vi "GUI_Bella_EnergyChart.vi"() -> ()   [LabVIEW 2013]
uses:
  Shared/GUI_Template/GUI_master/tcp_new_data_event.ctl
  Shared/GUI_Template/GUI_master/tcp new data cluster.ctl
panel:
  out "Numeric 2":dbl format="%#_4g"
  out "Numeric":dbl format="%#_4g"
  out "Numeric 4":dbl format="%#_4g"
  out "Numeric 3":dbl format="%#_4g"
  out "Numeric 7":dbl format="%#_4g"
  out "Numeric 9":dbl format="%#_4g"
  out "Numeric 5":dbl format="%#_4g"
  out "Numeric 6":dbl format="%#_4g"
  out "Numeric 8":dbl format="%#_4g"
  out "Numeric 10":dbl format="%#_4g"
  out "Numeric 11":dbl format="%#_4g"
  out "Numeric 12":dbl format="%#_4g"
  out "Numeric 13":dbl format="%#_4g"
  out "Numeric 14":dbl format="%#_4g"
  in  "stop":bool
  in  "RawField::1":dbl=0.001 caption="Raw Field" min=0.0 max=0.0 format="%_4f"
  in  "field::1":dbl=0.001 caption="Field" min=0.0 max=0.0 format="%_4p"
  in  "GUIdevice 1":string="BELLA_HallProbe"
  out "tcp data event":T1
  out "error IO 2":errorcluster
  # "Energy Chart"
  # "cam1"
  # "cam2"
  # "High Energy screen"
  # "[MeV/c]"
  # "Mid Energy screen"
  # "cam3"
  # "cam4"
  # "cam5"
  # "[MeV/c]"
  # "cam6"
  # "cam7"
  # "cam8"
  # "cam9"
  # "cam10"
  # "cam11"
  # "cam12"
  # "[MeV/c]"
  # "Low Energy screen, cam6 - 12"
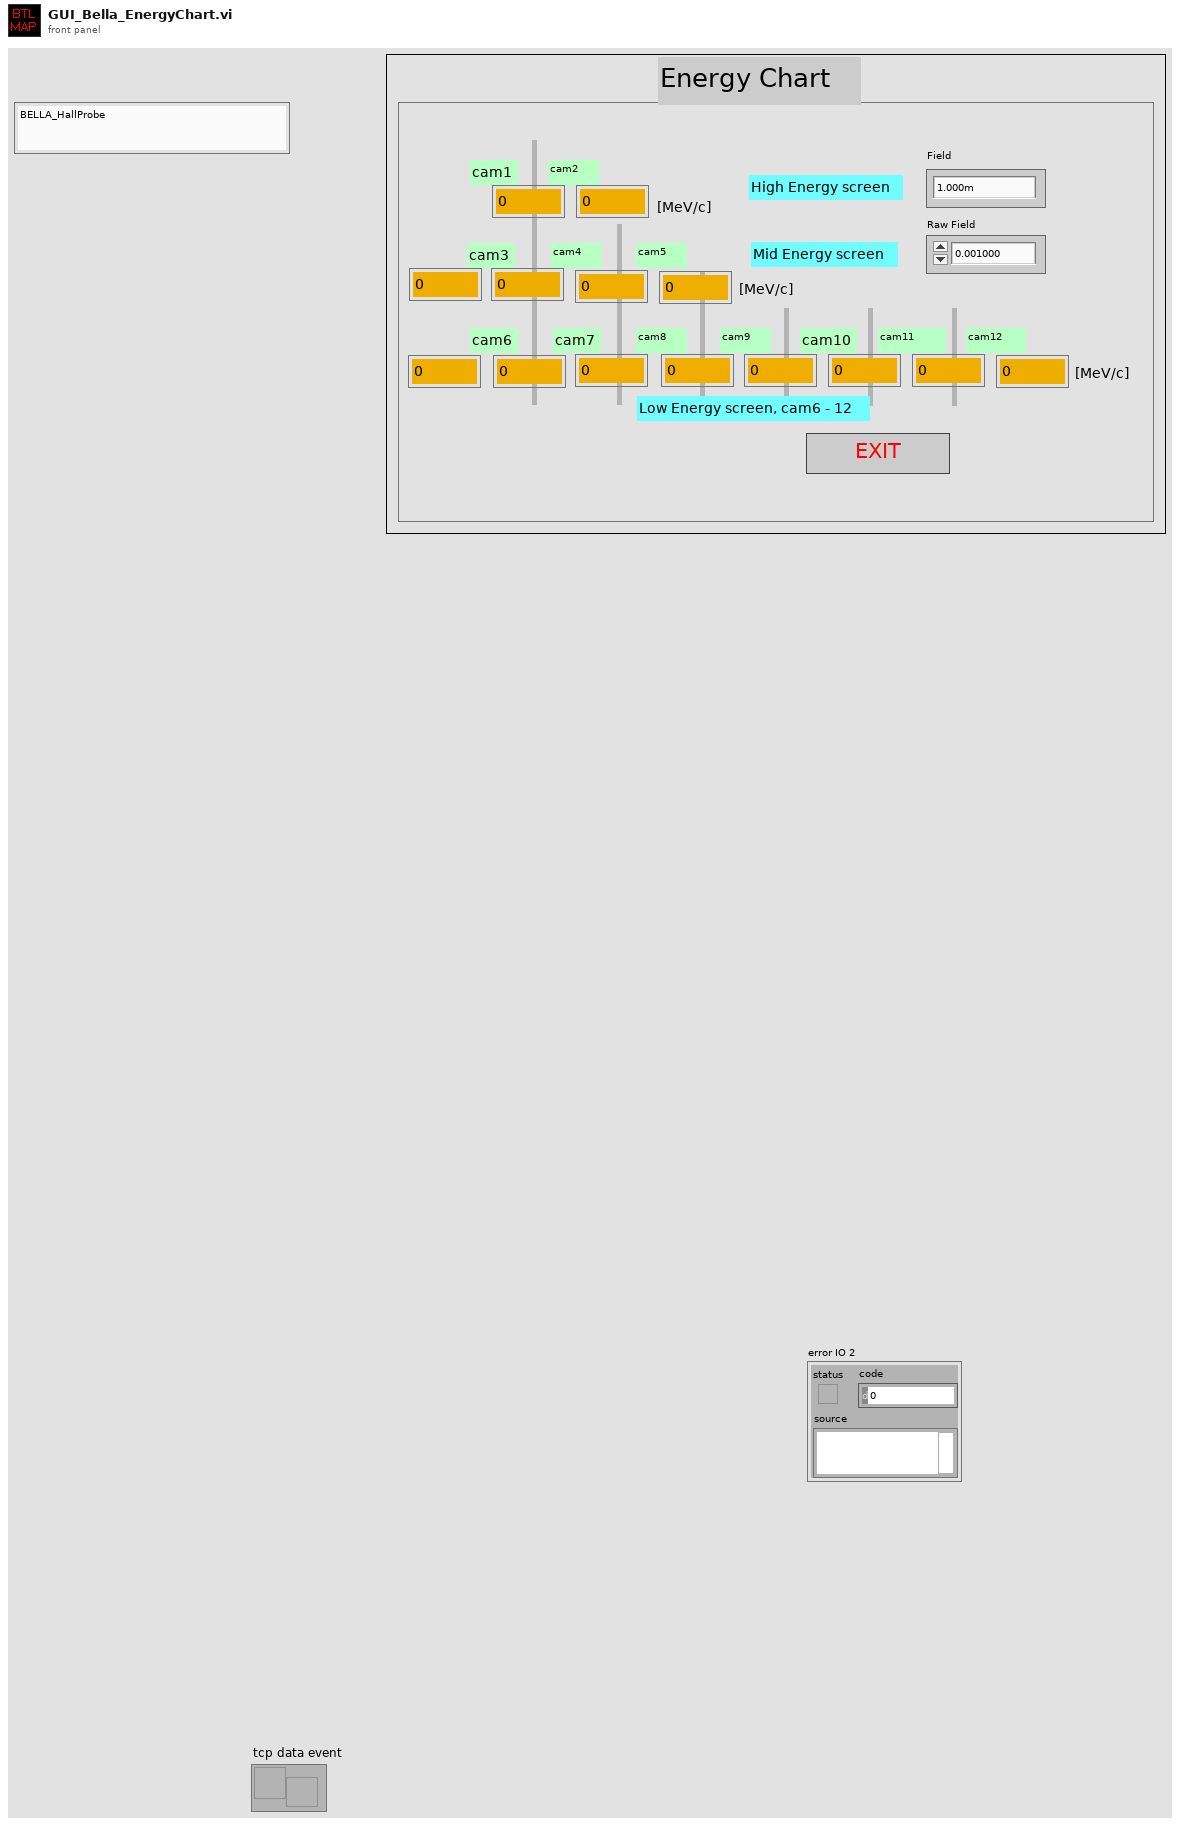
[diagram p1: front panel]
types:
  T1 = typedef "tcp_new_data_event.ctl" = refnum<user-event>
  T2 = typedef "tcp new data cluster.ctl" = cluster{"EventEnum":enum16{"new data", "connection status update"}, "Device name":string}
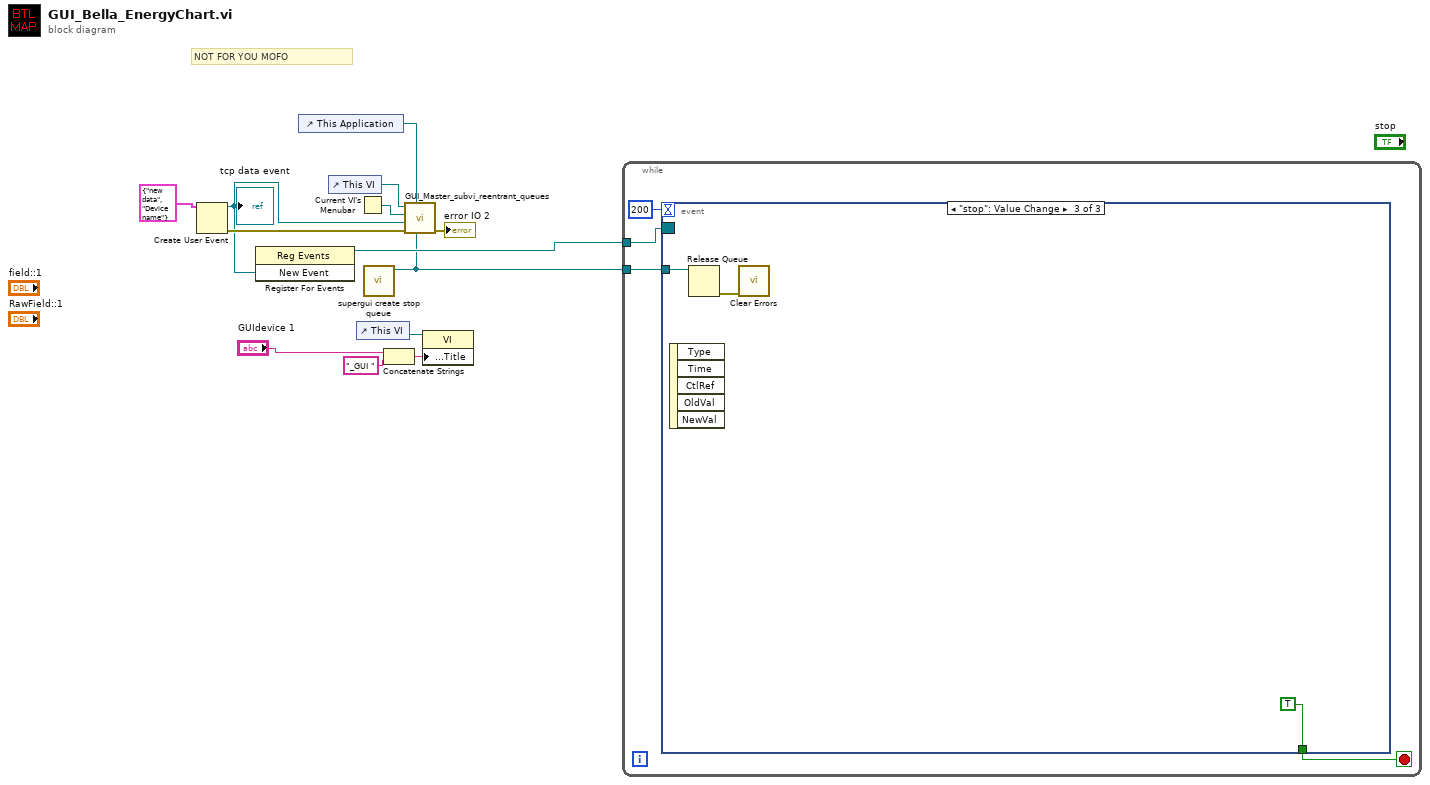
[diagram p0: block diagram]
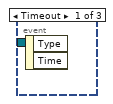
[diagram p2: hidden frame]
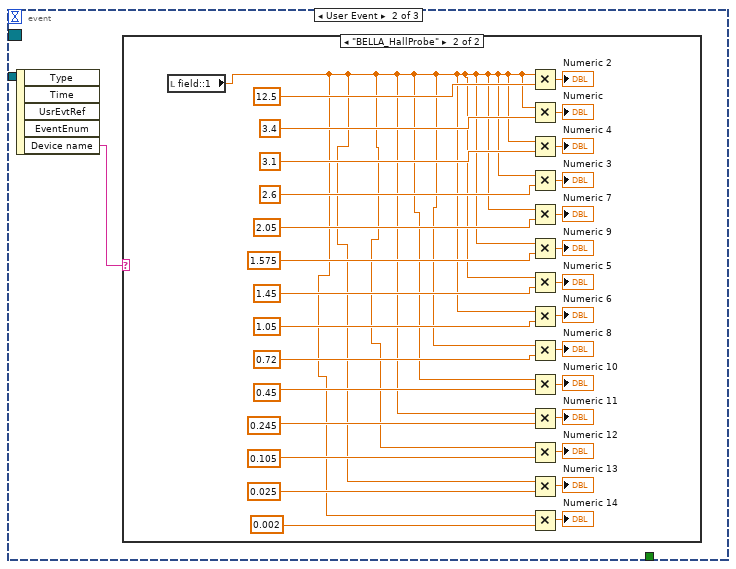
[diagram p3: hidden frame]
diagram:
  # "NOT FOR YOU MOFO"
  n1 = Create User Event(user event datatype=T2 {"EventEnum"=enum."new data", "Device name"="Device name"} ("New Event")) -> (user event=w8:refnum<user-event>, error out=w9:errorcluster)  [unwired: 1 in]
  "tcp data event" <- w8
  n2 = register-events(w8) -> (reference out=w6:refnum<event-registration>)  [unwired: 2 in, 1 out]
  n3 = control-ref of="This Application"() -> (w7:refnum<vi>)
  n4 = control-ref of="This VI"() -> (w12:refnum<vi>)
  n5 = control-ref of="This VI"() -> (w4:refnum<vi>)
  n6 = Current VI's Menubar() -> (w11:refnum<k9>)
  n7 = call "supergui create stop queue.vi"() -> ("STOP Queue out"=w5:refnum<queue>)  [unwired: 11 in]
  n8 = Concatenate Strings("GUIdevice 1", "_GUI ") -> (w3:string)
  n9 = call "GUI_Master_subvi_reentrant_queues.vi"("STOP Queue in"=w5, "This Application"=w7, "error in (no error)"=w9, "tcp data event"=w8, "Caller menu reference"=w11, "Caller VI ref"=w12) -> ("error out"=→"error IO 2":errorcluster)  [unwired: 5 in]
  n10 = property class="VI"(reference=w4, "Front Panel.Title"=w3) -> ()  [unwired: 1 in, 2 out]
  n11 = while {
    tunnel: w6 -> [w17]
    tunnel: w5 -> [w14]
    stop <- w16 stop-if-true
    n12 = event shown="[2] \"stop\": Value Change" {
      selector: w17 -> [_ _ _]
      dyn-events: _ -> [_ _ _]
      timeout: 200 -> [_ _ _]
      tunnel: [_ _ TRUE] -> w16
      tunnel: w14 -> [_ _ w49]
      event Timeout {
        n13 = event-data() -> ()  [unwired: 1 in, 2 out]
      }
      event User Event {
        n14 = event-data() -> ("Device name"=w18:string)  [unwired: 1 in, 4 out]
        n15 = case shown="\"BELLA_HallProbe\"" w18 {
          frame "False", Default {
          }
          frame "BELLA_HallProbe" {
            n16 = local read "field::1"() -> (w19:dbl)
            n17 = Multiply(x=w19, y=12.5) -> (x*y=→"Numeric 2":dbl)
            n18 = Multiply(x=w19, y=3.4) -> (x*y=→"Numeric":dbl)
            n19 = Multiply(x=w19, y=3.1) -> (x*y=→"Numeric 4":dbl)
            n20 = Multiply(x=w19, y=2.6) -> (x*y=→"Numeric 3":dbl)
            n21 = Multiply(x=w19, y=2.05) -> (x*y=→"Numeric 7":dbl)
            n22 = Multiply(x=w19, y=1.575) -> (x*y=→"Numeric 9":dbl)
            n23 = Multiply(x=w19, y=1.45) -> (x*y=→"Numeric 5":dbl)
            n24 = Multiply(x=w19, y=1.05) -> (x*y=→"Numeric 6":dbl)
            n25 = Multiply(x=w19, y=0.72) -> (x*y=→"Numeric 8":dbl)
            n26 = Multiply(x=w19, y=0.45) -> (x*y=→"Numeric 10":dbl)
            n27 = Multiply(x=w19, y=0.245) -> (x*y=→"Numeric 11":dbl)
            n28 = Multiply(x=w19, y=0.105) -> (x*y=→"Numeric 12":dbl)
            n29 = Multiply(x=w19, y=0.025) -> (x*y=→"Numeric 13":dbl)
            n30 = Multiply(x=w19, y=0.002) -> (x*y=→"Numeric 14":dbl)
          }
        }
      }
      event "stop": Value Change {
        n31 = event-data() -> ()  [unwired: 1 in, 5 out]
        n32 = Release Queue(queue=w49) -> (error out=w48:errorcluster)  [unwired: 2 in, 2 out]
        n33 = call <vilib>:"Clear Errors.vi"("error in (no error)"=w48) -> ()  [unwired: 6 in, 1 out]
      }
    }
  }
